vi "空载试验判定.vi"(7 "Result":refnum<vi>, 10 "判定参数":T1, 11 "XY曲线":cluster{"X":dbl[], "Y":dbl[]}[](array[cluster])) -> (2 "判定项长度":i32, 3 "OK？":bool)   [LabVIEW 2020]
uses:
  <userlib>/_MGI/1D Array/MGI Average/MGI Average (DBL[]).vi
panel:
  out "逆向平均值":dbl
  out "正向平均值":dbl
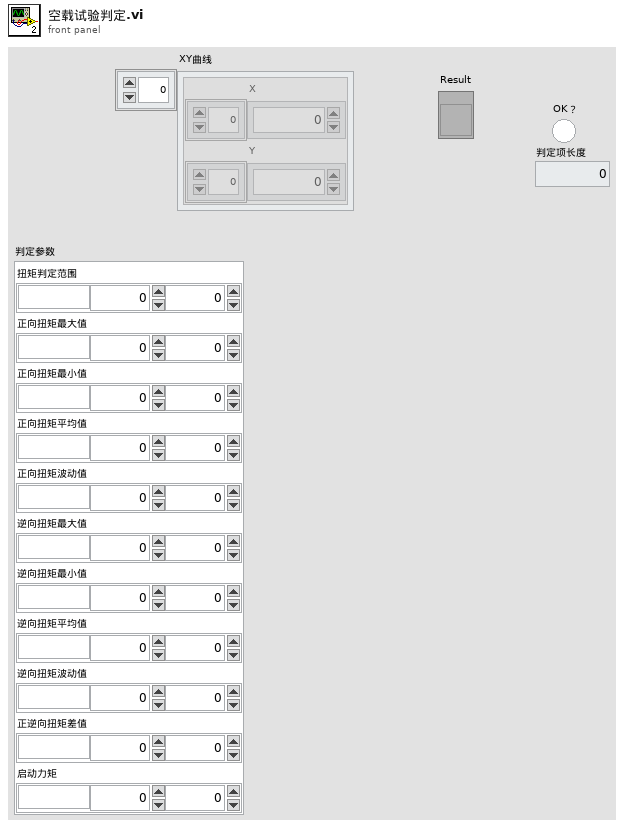
[diagram p1: front panel]
types:
  T1 = cluster{"扭矩判定范围":cluster{"单位":string, "下限":dbl, "上限":dbl}, "正向扭矩最大值":cluster{"单位":string, "下限":dbl, "上限":dbl}, "正向扭矩最小值":cluster{"单位":string, "下限":dbl, "上限":dbl}, "正向扭矩平均值":cluster{"单位":string, "下限":dbl, "上限":dbl}, "正向扭矩波动值":cluster{"单位":string, "下限":dbl, "上限":dbl}, "逆向扭矩最大值":cluster{"单位":string, "下限":dbl, "上限":dbl}, "逆向扭矩最小值":cluster{"单位":string, "下限":dbl, "上限":dbl}, "逆向扭矩平均值":cluster{"单位":string, "下限":dbl, "上限":dbl}, "逆向扭矩波动值":cluster{"单位":string, "下限":dbl, "上限":dbl}, "正逆向扭矩差值":cluster{"单位":string, "下限":dbl, "上限":dbl}, "启动力矩":cluster{"单位":string, "下限":dbl, "上限":dbl}}
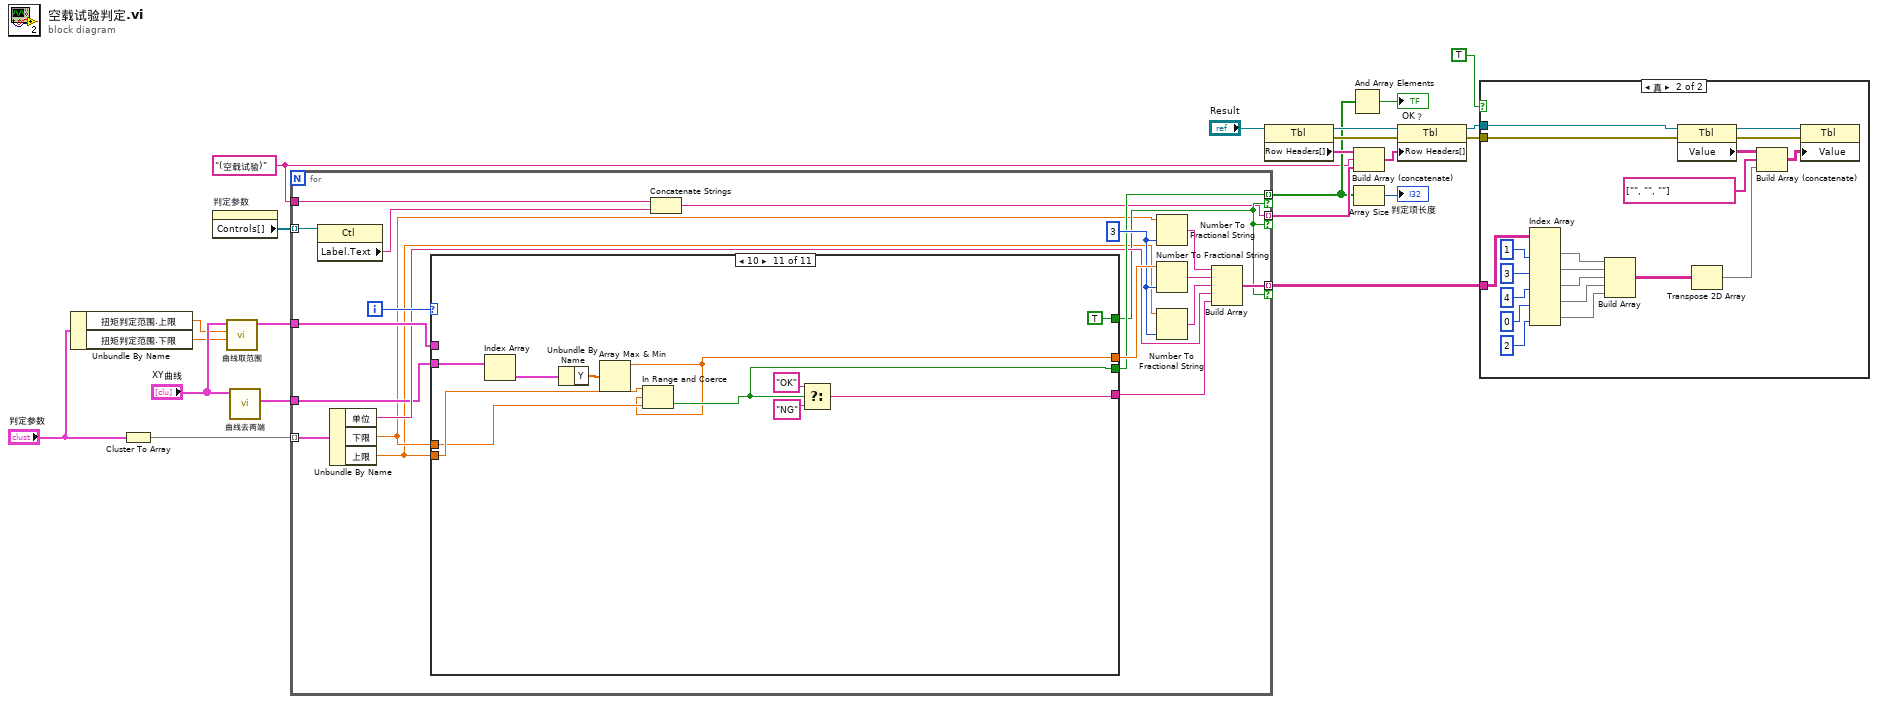
[diagram p0: block diagram]
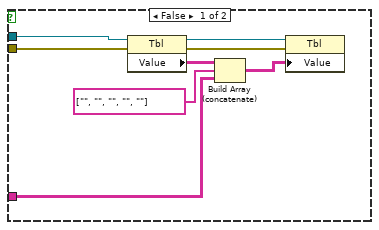
[diagram p2: hidden frame]
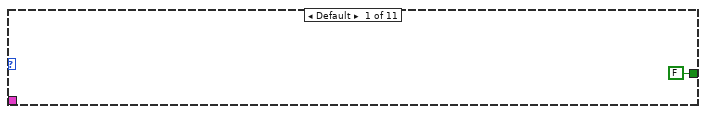
[diagram p3: hidden frame]
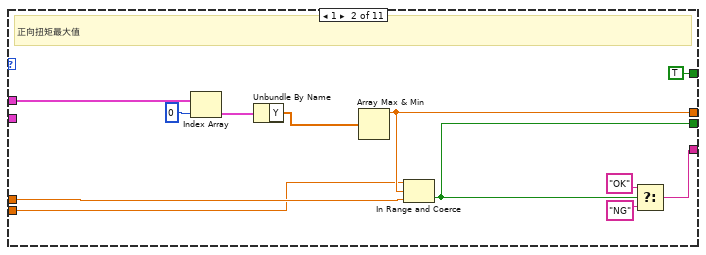
[diagram p4: hidden frame]
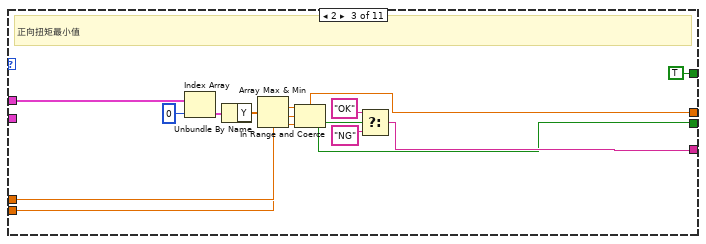
[diagram p5: hidden frame]
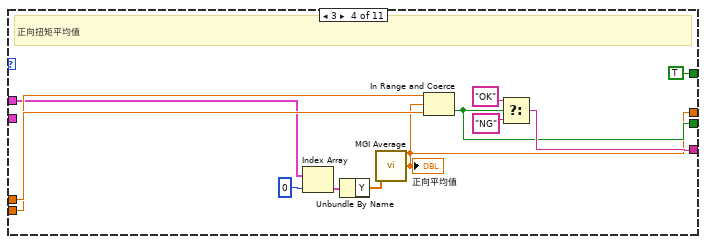
[diagram p6: hidden frame]
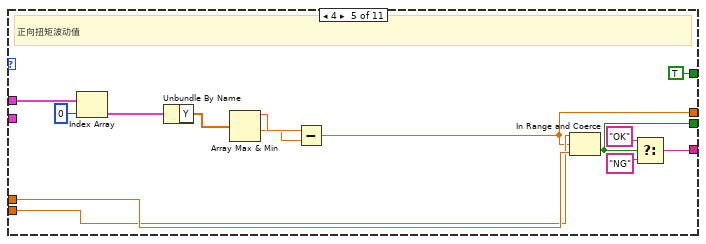
[diagram p7: hidden frame]
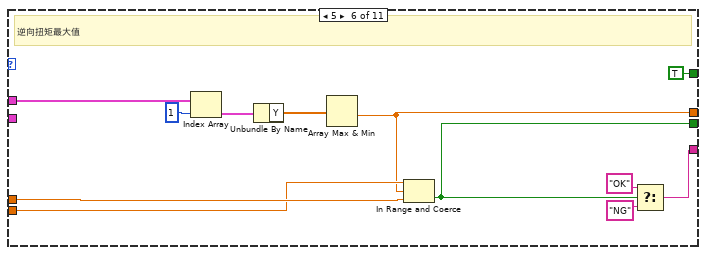
[diagram p8: hidden frame]
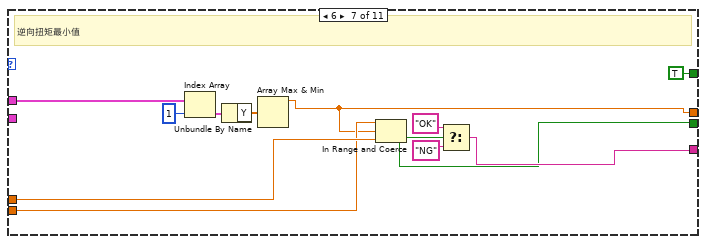
[diagram p9: hidden frame]
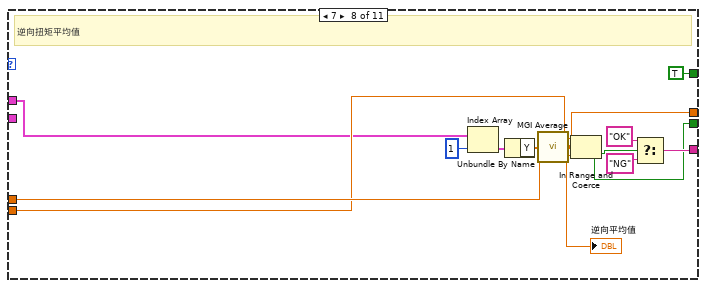
[diagram p10: hidden frame]
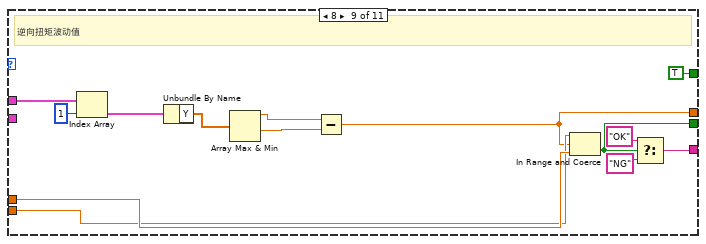
[diagram p11: hidden frame]
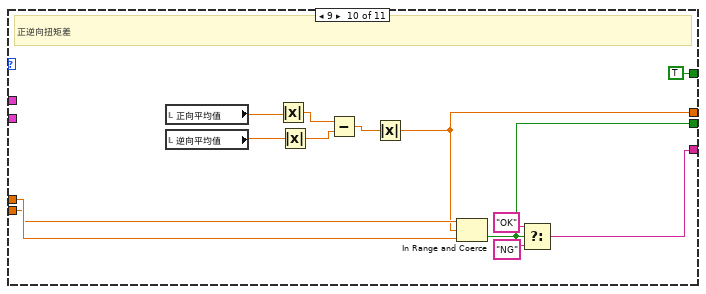
[diagram p12: hidden frame]
diagram:
  w6 = "(空载试验)" ("Label.Text")
  n1 = Unbundle By Name("判定参数") -> ("扭矩判定范围.上限"=w2:dbl, "扭矩判定范围.下限"=w1:dbl)
  n2 = Cluster To Array(cluster="判定参数") -> (array=w22:cluster{"单位":string, "下限":dbl, "上限":dbl}[])
  n3 = property on="判定参数" class="Clust (严格)"() -> ("Controls[]"=w11:refnum<vi>[])  [unwired: 2 in, 2 out]
  n4 = call "曲线取范围.vi"("下限"=w1, "上限"=w2, "曲线In"="XY曲线") -> ("曲线Out"=w4:cluster{"X":dbl[], "Y":dbl[]}[])  [unwired: 8 in]
  n5 = call "曲线去两端.vi"("曲线In"="XY曲线") -> ("启动曲线"=w7:cluster{"X":dbl[], "Y":dbl[]}[])  [unwired: 9 in, 1 out]
  n6 = for {
    tunnel: w22 -> [w42] mode=indexing
    tunnel: w11 -> [w40] mode=indexing
    tunnel: w4 -> [w38]
    tunnel: [w32] -> w9 mode=indexing if=w28
    tunnel: [w30] -> w12 mode=indexing if=w28
    tunnel: [w24] -> w15 mode=indexing if=w28
    tunnel: w7 -> [w27]
    tunnel: w6 -> [w23]
    i -> [w41]
    w37 = i16 3 ("精度(6)")
    n7 = property class="Ctl"(reference=w40) -> ("Label.Text"=w29:string)  [unwired: 1 in, 2 out]
    n8 = Unbundle By Name(w42) -> ("单位"=w31:string, "下限"=w26:dbl, "上限"=w25:dbl)
    n9 = case shown="10" w41 {
      tunnel: [_ w52 w58 w69 w80 w94 w106 w118 w130 w144 w158] -> w39
      tunnel: w38 -> [_ w55 w67 w72 w86 w105 w117 w122 w136 _ _]
      tunnel: [_ w49 w63 w77 w91 w100 w113 w127 w141 w146 w157] -> w33
      tunnel: [_ w48 w62 w76 w90 w99 w112 w126 w140 w145 w159] -> w32
      tunnel: w26 -> [_ w47 w61 w75 w89 w98 w111 w125 w139 w153 w163]
      tunnel: w25 -> [_ w46 w60 w74 w88 w97 w110 w124 w138 w152 w164]
      tunnel: [FALSE TRUE TRUE TRUE TRUE TRUE TRUE TRUE TRUE TRUE TRUE] -> w28
      tunnel: w27 -> [_ _ _ _ _ _ _ _ _ _ w167]
      frame Default {
      }
      frame 1 {
        # "正向扭矩最大值"
        n10 = Index Array(array=w55, index=0 ("索引")) -> (element=w53:cluster{"X":dbl[], "Y":dbl[]})
        n11 = Unbundle By Name(w53) -> ("Y"=w44:dbl[])
        n12 = Array Max & Min(array=w44) -> (max value=w52:dbl)  [unwired: 3 out]
        n13 = In Range and Coerce(upper limit=w46, x=w52, lower limit=w47) -> (In Range?=w48:bool)  [unwired: 1 out]
        n14 = Select(t="OK", s=w48, f="NG") -> (s? t:f=w49:string)
      }
      frame 2 {
        # "正向扭矩最小值"
        n15 = Index Array(array=w67, index=0 ("索引")) -> (element=w66:cluster{"X":dbl[], "Y":dbl[]})
        n16 = Unbundle By Name(w66) -> ("Y"=w57:dbl[])
        n17 = Array Max & Min(array=w57) -> (min value=w58:dbl)  [unwired: 3 out]
        n18 = In Range and Coerce(upper limit=w60, x=w58, lower limit=w61) -> (In Range?=w62:bool)  [unwired: 1 out]
        n19 = Select(t="OK", s=w62, f="NG") -> (s? t:f=w63:string)
      }
      frame 3 {
        # "正向扭矩平均值"
        n20 = Index Array(array=w72, index=0 ("索引")) -> (element=w71:cluster{"X":dbl[], "Y":dbl[]})
        n21 = Unbundle By Name(w71) -> ("Y"=w68:dbl[])
        n22 = call-poly <userlib>:"MGI Average.vi"("Double[]"=w68) -> ("Average"=w69:dbl)  [unwired: 1 in]
        "正向平均值" <- w69
        n23 = In Range and Coerce(upper limit=w74, x=w69, lower limit=w75) -> (In Range?=w76:bool)  [unwired: 1 out]
        n24 = Select(t="OK", s=w76, f="NG") -> (s? t:f=w77:string)
      }
      frame 4 {
        # "正向扭矩波动值"
        n25 = Index Array(array=w86, index=0 ("索引")) -> (element=w85:cluster{"X":dbl[], "Y":dbl[]})
        n26 = Unbundle By Name(w85) -> ("Y"=w83:dbl[])
        n27 = Array Max & Min(array=w83) -> (max value=w82:dbl, min value=w81:dbl)  [unwired: 2 out]
        n28 = Subtract(x=w82, y=w81) -> (x-y=w80:dbl)
        n29 = In Range and Coerce(upper limit=w88, x=w80, lower limit=w89) -> (In Range?=w90:bool)  [unwired: 1 out]
        n30 = Select(t="OK", s=w90, f="NG") -> (s? t:f=w91:string)
      }
      frame 5 {
        # "逆向扭矩最大值"
        n31 = Index Array(array=w105, index=1 ("索引")) -> (element=w103:cluster{"X":dbl[], "Y":dbl[]})
        n32 = Unbundle By Name(w103) -> ("Y"=w95:dbl[])
        n33 = Array Max & Min(array=w95) -> (min value=w94:dbl)  [unwired: 3 out]
        n34 = In Range and Coerce(upper limit=w97, x=w94, lower limit=w98) -> (In Range?=w99:bool)  [unwired: 1 out]
        n35 = Select(t="OK", s=w99, f="NG") -> (s? t:f=w100:string)
      }
      frame 6 {
        # "逆向扭矩最小值"
        n36 = Index Array(array=w117, index=1 ("索引")) -> (element=w116:cluster{"X":dbl[], "Y":dbl[]})
        n37 = Unbundle By Name(w116) -> ("Y"=w108:dbl[])
        n38 = Array Max & Min(array=w108) -> (max value=w106:dbl)  [unwired: 3 out]
        n39 = In Range and Coerce(upper limit=w110, x=w106, lower limit=w111) -> (In Range?=w112:bool)  [unwired: 1 out]
        n40 = Select(t="OK", s=w112, f="NG") -> (s? t:f=w113:string)
      }
      frame 7 {
        # "逆向扭矩平均值"
        n41 = Index Array(array=w122, index=1 ("索引")) -> (element=w121:cluster{"X":dbl[], "Y":dbl[]})
        n42 = Unbundle By Name(w121) -> ("Y"=w120:dbl[])
        n43 = call-poly <userlib>:"MGI Average.vi"("Double[]"=w120) -> ("Average"=w118:dbl)  [unwired: 1 in]
        "逆向平均值" <- w118
        n44 = In Range and Coerce(upper limit=w124, x=w118, lower limit=w125) -> (In Range?=w126:bool)  [unwired: 1 out]
        n45 = Select(t="OK", s=w126, f="NG") -> (s? t:f=w127:string)
      }
      frame 8 {
        # "逆向扭矩波动值"
        n46 = Index Array(array=w136, index=1 ("索引")) -> (element=w135:cluster{"X":dbl[], "Y":dbl[]})
        n47 = Unbundle By Name(w135) -> ("Y"=w133:dbl[])
        n48 = Array Max & Min(array=w133) -> (max value=w132:dbl, min value=w131:dbl)  [unwired: 2 out]
        n49 = Subtract(x=w132, y=w131) -> (x-y=w130:dbl)
        n50 = In Range and Coerce(upper limit=w138, x=w130, lower limit=w139) -> (In Range?=w140:bool)  [unwired: 1 out]
        n51 = Select(t="OK", s=w140, f="NG") -> (s? t:f=w141:string)
      }
      frame 9 {
        # "正逆向扭矩差"
        n52 = local read "正向平均值"() -> (w151:dbl)
        n53 = local read "逆向平均值"() -> (w150:dbl)
        n54 = Absolute Value(x=w151) -> (abs(x)=w149:dbl)
        n55 = Absolute Value(x=w150) -> (abs(x)=w148:dbl)
        n56 = Subtract(x=w149, y=w148) -> (x-y=w147:dbl)
        n57 = Absolute Value(x=w147) -> (abs(x)=w144:dbl)
        n58 = In Range and Coerce(upper limit=w152, x=w144, lower limit=w153) -> (In Range?=w145:bool)  [unwired: 1 out]
        n59 = Select(t="OK", s=w145, f="NG") -> (s? t:f=w146:string)
      }
      frame 10 {
        n60 = Index Array(array=w167) -> (element=w166:cluster{"X":dbl[], "Y":dbl[]})  [unwired: 1 in]
        n61 = Unbundle By Name(w166) -> ("Y"=w165:dbl[])
        n62 = Array Max & Min(array=w165) -> (max value=w158:dbl)  [unwired: 3 out]
        n63 = In Range and Coerce(upper limit=w164, x=w158, lower limit=w163) -> (In Range?=w159:bool)  [unwired: 1 out]
        n64 = Select(t="OK", s=w159, f="NG") -> (s? t:f=w157:string)
      }
    }
    n65 = Concatenate Strings(w23, w29) -> (w24:string)
    n66 = Number To Fractional String(number=w26, precision (6)=w37) -> (F-format string=w36:string)  [unwired: 2 in]
    n67 = Number To Fractional String(number=w39, precision (6)=w37) -> (F-format string=w35:string)  [unwired: 2 in]
    n68 = Number To Fractional String(number=w25, precision (6)=w37) -> (F-format string=w34:string)  [unwired: 2 in]
    n69 = Build Array(w36, w35, w34, w31, w33) -> (w30:string[])
  }
  n70 = property class="Tbl"(reference="Result") -> (reference out=w17:refnum<vi>, error out=w20:errorcluster, "Row Headers[]"=w13:string[])  [unwired: 1 in]
  n71 = And Array Elements(Boolean array=w9) -> (logical AND=→"OK？":bool)
  n72 = Build Array (concatenate)(w13, w6, w15) -> (w16:string[])
  n73 = Array Size(array=w9) -> (size(s)=→"判定项长度":i32)
  n74 = property class="Tbl"(reference=w17, error in=w20, "Row Headers[]"=w16) -> (reference out=w18:refnum<vi>, error out=w19:errorcluster)
  n75 = case shown="真" TRUE {
    tunnel: w19 -> [w173 w193]
    tunnel: w18 -> [w170 w190]
    tunnel: w12 -> [w169 w188]
    frame False {
      n76 = property class="Tbl"(reference=w170, error in=w173) -> (reference out=w171:refnum<vi>, error out=w172:errorcluster, "Value"=w174:string[][])
      n77 = Build Array (concatenate)(w174, string[] ["", "", "", "", ""], w169) -> (w175:string[][])
      n78 = property class="Tbl"(reference=w171, error in=w172, "Value"=w175) -> ()  [unwired: 2 out]
    }
    frame True {
      n79 = Index Array(array=w188, index (col) #1=1 ("禁用的索引 (列)"), index (col) #2=3 ("索引 (列)"), index (col) #3=4 ("索引 (列)"), index (col) #4=0 ("索引 (列)"), index (col) #5=2 ("索引 (列)")) -> (element #1=w184:string[], element #2=w183:string[], element #3=w182:string[], element #4=w177:string[], element #5=w176:string[])  [unwired: 5 in]
      n80 = Build Array(w184, w183, w182, w177, w176) -> (w181:string[][])
      n81 = property class="Tbl"(reference=w190, error in=w193) -> (reference out=w191:refnum<vi>, error out=w192:errorcluster, "Value"=w194:string[][])
      n82 = Transpose 2D Array(2D array=w181) -> (transposed array=w180:string[][])
      n83 = Build Array (concatenate)(w194, string[] ["", "", ""], w180) -> (w195:string[][])
      n84 = property class="Tbl"(reference=w191, error in=w192, "Value"=w195) -> ()  [unwired: 2 out]
    }
  }
